vi "Cache INI Section--constant.vi"() -> (3 "Cache INI Section":string)   [LabVIEW 2025]
doc: "Section name for Cache File"
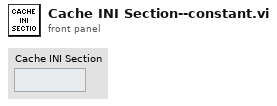
[diagram p1: front panel]
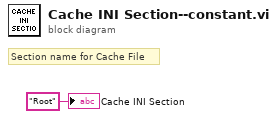
[diagram p0: block diagram]
diagram:
  # "Section name for Cache File"
  "Cache INI Section" <- "Root" ("Fallback INI Section")
